vi "DriveStateController.vi"(0 "Vertical_Throttle":dbl, 2 "Lateral_Throttle":dbl, 5 "Rotational_Throttle":dbl) -> (12 "Drive_Motor_Front_Right":dbl, 13 "Azimuth_Motor_Back_Right":dbl, 14 "Drive_Motor_Front_Left":dbl, 15 "Drive_Motor_Back_Left":dbl, 16 "Drive_Motor_Back_Right":dbl, 17 "Azimuth_Motor_Front_Right":dbl, 18 "Azimuth_Motor_Front_Left":dbl, 19 "Azimuth_Motor_Back_Left":dbl)   [LabVIEW 2019]
uses:
  Globals/Sensor_Values.vi
panel:
  in  "Deadband":dbl=0.1
  in  "Hysteresis (deg)":dbl=20.0 format="%#_13g"
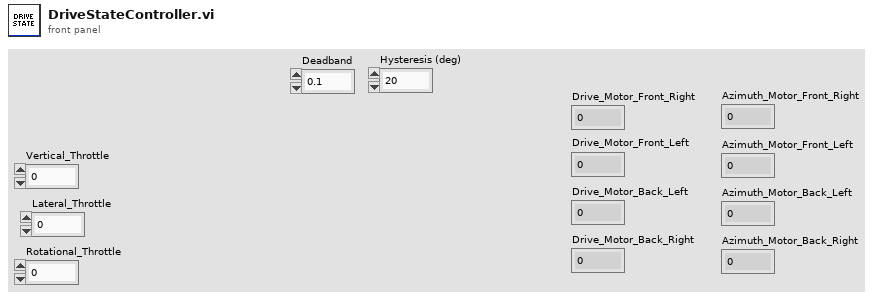
[diagram p1: front panel]
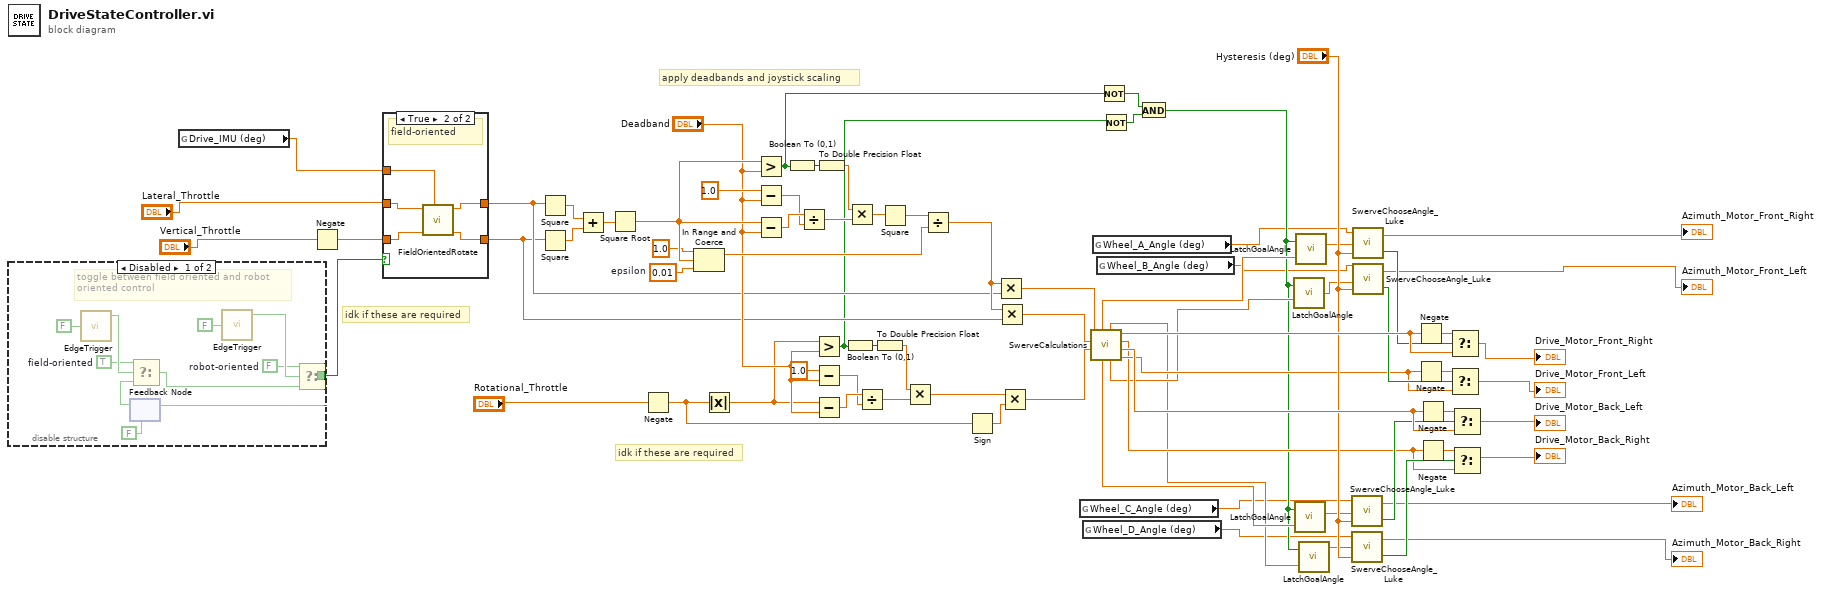
[diagram p0: block diagram]
diagram:
  w53 = 0.01  # epsilon
  # "idk if these are required"
  # "idk if these are required"
  # "apply deadbands and joystick scaling"
  n1 = disable-structure shown="Disabled" {
    disable-tunnel: [w86 _] -> w37
    frame Disabled {
      w81 = TRUE  # field-oriented
      w83 = FALSE  # robot-oriented
      # "toggle between field oriented and robot \noriented control"
      n2 = call "EdgeTrigger.vi"("Input Signal"=FALSE) -> ("Rising Edge Trigger"=w82:bool)  [unwired: 2 out]
      n3 = feedback #1(FALSE) -> (w79:bool)
      n4 = Select(t=w81, s=w82, f=w79) -> (s? t:f=w80:bool)
      n5 = call "EdgeTrigger.vi"("Input Signal"=FALSE) -> ("Rising Edge Trigger"=w84:bool)  [unwired: 2 out]
      n6 = Select(t=w83, s=w84, f=w80) -> (s? t:f=w86:bool)
      n7 = feedback-in #1(w86) -> ()
    }
    frame Enabled {
    }
  }
  n8 = global read "Sensor_Values.vi" "Drive_IMU (deg)"() -> (w5:dbl)
  n9 = Negate(x="Vertical_Throttle") -> (-x=w39:dbl)
  n10 = case shown="True" w37 {
    tunnel: [w88 w93] -> w40
    tunnel: "Lateral_Throttle" -> [w88 w91]
    tunnel: [w87 w92] -> w38
    tunnel: w39 -> [w87 w90]
    tunnel: w5 -> [_ w89]
    frame False {
      # "robot-oriented"
    }
    frame True {
      # "field-oriented"
      n11 = call "FieldOrientedRotate.vi"("Angle (deg)"=w89, "Y"=w90, "X"=w91) -> ("Y'"=w92:dbl, "X'"=w93:dbl)  [unwired: 7 in]
    }
  }
  n12 = Square(x=w40) -> (x^2=w57:dbl)
  n13 = Square(x=w38) -> (x^2=w58:dbl)
  n14 = Add(x=w57, y=w58) -> (x+y=w56:dbl)
  n15 = Square Root(x=w56) -> (sqrt(x)=w52:dbl)
  n16 = Negate(x="Rotational_Throttle") -> (-x=w31:dbl)
  n17 = In Range and Coerce(upper limit=1.0, x=w52, lower limit=w53) -> (coerced(x)=w54:dbl)  [unwired: 1 out]
  n18 = Absolute Value(x=w31) -> (abs(x)=w34:dbl)
  n19 = Greater?(x=w52, y="Deadband") -> (0:w27:bool)
  n20 = Subtract(x=1.0, y="Deadband") -> (x-y=w60:dbl)
  n21 = Subtract(x=w52, y="Deadband") -> (x-y=w62:dbl)
  n22 = Boolean To (0,1)(Boolean=w27) -> (0, 1=w65:i16)
  n23 = Divide(x=w62, y=w60) -> (x/y=w59:dbl)
  n24 = Greater?(x=w34, y="Deadband") -> (0:w26:bool)
  n25 = Subtract(x=1.0, y="Deadband") -> (x-y=w43:dbl)
  n26 = Subtract(x=w34, y="Deadband") -> (x-y=w45:dbl)
  n27 = To Double Precision Float(number=w65) -> (double precision float=w64:dbl)
  n28 = Boolean To (0,1)(Boolean=w26) -> (0, 1=w47:i16)
  n29 = Multiply(x=w64, y=w59) -> (x*y=w63:dbl)
  n30 = Divide(x=w45, y=w43) -> (x/y=w42:dbl)
  n31 = To Double Precision Float(number=w47) -> (double precision float=w46:dbl)
  n32 = Square(x=w63) -> (x^2=w55:dbl)
  n33 = Multiply(x=w46, y=w42) -> (x*y=w30:dbl)
  n34 = Divide(x=w55, y=w54) -> (x/y=w50:dbl)
  n35 = Sign(1:w31) -> (0:w35:dbl)
  n36 = Multiply(x=w50, y=w40) -> (x*y=w49:dbl)
  n37 = Multiply(x=w50, y=w38) -> (x*y=w48:dbl)
  n38 = Multiply(x=w30, y=w35) -> (x*y=w36:dbl)
  n39 = global read "Sensor_Values.vi" "Wheel_C_Angle (deg)"() -> (w2:dbl)
  n40 = global read "Sensor_Values.vi" "Wheel_D_Angle (deg)"() -> (w1:dbl)
  n41 = call "SwerveCalculations.vi"("j2x"=w36, "j1y"=w48, "j1x"=w49) -> ("magnitude4"=w33:dbl, "magnitude3"=w75:dbl, "magnitude2"=w32:dbl, "magnitude1"=w74:dbl, "Wheel Angle4"=w23:dbl, "Wheel Angle2"=w18:dbl, "Wheel Angle3"=w21:dbl, "wheel angle 1"=w29:dbl)  [unwired: 1 in]
  n42 = global read "Sensor_Values.vi" "Wheel_A_Angle (deg)"() -> (w4:dbl)
  n43 = global read "Sensor_Values.vi" "Wheel_B_Angle (deg)"() -> (w3:dbl)
  n44 = Not(x=w27) -> (.not. x?=w24:bool)
  n45 = Not(x=w26) -> (.not. x?=w25:bool)
  n46 = And(x=w24, y=w25) -> (x .and. y?=w17:bool)
  n47 = call "LatchGoalAngle.vi"("Raw Goal Angle"=w23, "In Deadband"=w17) -> ("Latched Goal Angle"=w22:dbl)
  n48 = call "LatchGoalAngle.vi"("Raw Goal Angle"=w21, "In Deadband"=w17) -> ("Latched Goal Angle"=w20:dbl)
  n49 = call "LatchGoalAngle.vi"("Raw Goal Angle"=w29, "In Deadband"=w17) -> ("Latched Goal Angle"=w28:dbl)
  n50 = call "LatchGoalAngle.vi"("Raw Goal Angle"=w18, "In Deadband"=w17) -> ("Latched Goal Angle"=w19:dbl)
  n51 = call "SwerveChooseAngle_Luke.vi"("Hysteresis (deg)"="Hysteresis (deg)", "Goal Angle (deg)"=w20, "Current Angle (deg)"=w2) -> ("Invert Speed  Motor (?)"=w72:bool, "Angular Distance (deg)"=→"Azimuth_Motor_Back_Left":dbl)
  n52 = call "SwerveChooseAngle_Luke.vi"("Hysteresis (deg)"="Hysteresis (deg)", "Goal Angle (deg)"=w19, "Current Angle (deg)"=w1) -> ("Invert Speed  Motor (?)"=w71:bool, "Angular Distance (deg)"=→"Azimuth_Motor_Back_Right":dbl)
  n53 = call "SwerveChooseAngle_Luke.vi"("Hysteresis (deg)"="Hysteresis (deg)", "Goal Angle (deg)"=w28, "Current Angle (deg)"=w4) -> ("Invert Speed  Motor (?)"=w68:bool, "Angular Distance (deg)"=→"Azimuth_Motor_Front_Right":dbl)
  n54 = call "SwerveChooseAngle_Luke.vi"("Hysteresis (deg)"="Hysteresis (deg)", "Goal Angle (deg)"=w22, "Current Angle (deg)"=w3) -> ("Invert Speed  Motor (?)"=w67:bool, "Angular Distance (deg)"=→"Azimuth_Motor_Front_Left":dbl)
  n55 = Negate(x=w74) -> (-x=w70:dbl)
  n56 = Negate(x=w33) -> (-x=w69:dbl)
  n57 = Negate(x=w75) -> (-x=w76:dbl)
  n58 = Negate(x=w32) -> (-x=w66:dbl)
  n59 = Select(t=w70, s=w68, f=w74) -> (s? t:f=→"Drive_Motor_Front_Right":dbl)
  n60 = Select(t=w69, s=w67, f=w33) -> (s? t:f=→"Drive_Motor_Front_Left":dbl)
  n61 = Select(t=w76, s=w72, f=w75) -> (s? t:f=→"Drive_Motor_Back_Left":dbl)
  n62 = Select(t=w66, s=w71, f=w32) -> (s? t:f=→"Drive_Motor_Back_Right":dbl)
